vi "Format Errors.vi"(8 "error in (no error)":errorcluster[](array[cluster]), 11 "Channel in":refnum<class "Channel.lvclass">) -> (0 "error out":errorcluster, 3 "Channel out":refnum<class "Channel.lvclass">)   [LabVIEW 2015, in "Channel.lvclass"]
uses:
  Channel.lvclass
  Channel.lvclass/Channel.ctl
  <vilib>/regexp/Match Regular Expression.xnode
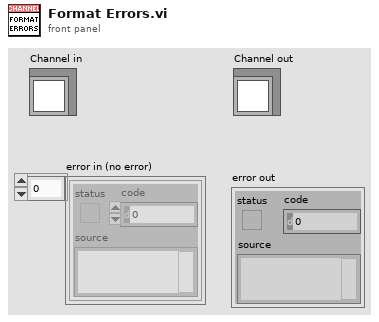
[diagram p1: front panel]
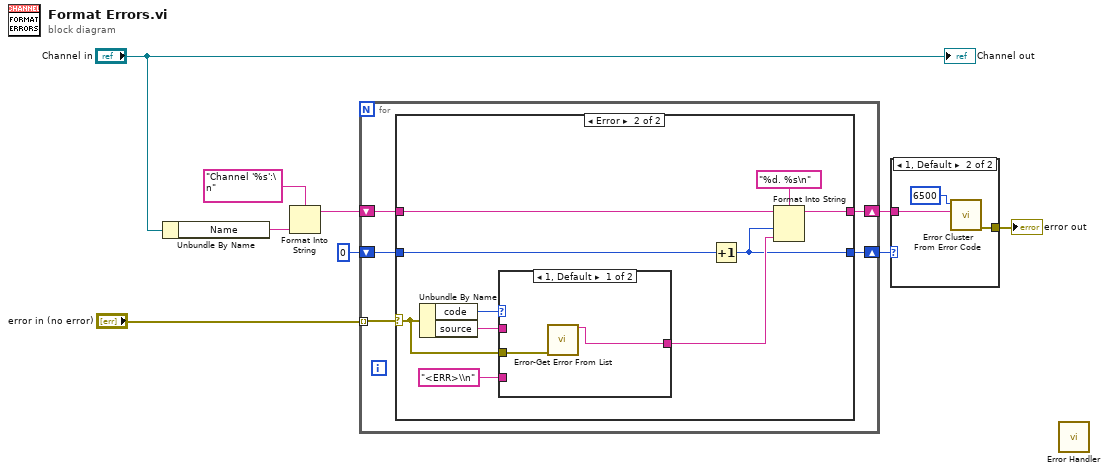
[diagram p0: block diagram]
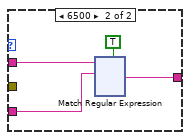
[diagram p4: hidden frame]
diagram:
  n1 = Unbundle By Name("Channel in") -> ("Name"=w6:string)
  n2 = Format Into String(format string="Channel '%s':\n", w6) -> (resulting string=w4:string)  [unwired: 2 in, 1 out]
  n3 = for {
    tunnel: "error in (no error)" -> [w12] mode=indexing
    shift-right: [w13] -> w3
    shift-left: w4 -> [w14]
    shift-right: [w11] -> w1
    shift-left: 0 -> [w10]
    n4 = case shown="Error" w12 {
      selector: w12 -> [_ w17]
      tunnel: w14 -> [w16 w26]
      tunnel: [w16 w25] -> w13
      tunnel: [w15 w19] -> w11
      tunnel: w10 -> [w15 w20]
      frame No Error {
      }
      frame Error {
        n5 = Unbundle By Name(w17) -> ("code"=w18:i32, "source"=w22:string)
        n6 = case shown="1, Default" w18 {
          tunnel: "<ERR>\\n" ("regular expression") -> [_ w31]
          tunnel: w22 -> [_ w30]
          tunnel: [w27 w29] -> w21
          tunnel: w17 -> [w28 _]
          frame 1, Default {
            n7 = call "Error-Get Error From List.vi"("error IO"=w28) -> ("Description"=w27:string)  [unwired: 11 in, 3 out]
          }
          frame 6500 {
            n8 = xnode "Match Regular Expression"("input string"=w30, "regular expression"=w31, "multiline? (F)"=TRUE) -> ("after match"=w29:string)  [unwired: 3 in, 4 out]
          }
        }
        n9 = Increment(x=w20) -> (x+1=w19:i32)
        n10 = Format Into String(format string="%d. %s\n", initial string=w26, w19, w21) -> (resulting string=w25:string)  [unwired: 1 in, 1 out]
      }
    }
  }
  n11 = case shown="1, Default" w1 {
    tunnel: [_ w149] -> w8
    tunnel: w3 -> [_ w148]
    frame 0 {
    }
    frame 1, Default {
      n12 = call <vilib>:"Error Cluster From Error Code.vi"("error message (\"\")"=w148, "error code (0)"=6500) -> ("error out"=w149:errorcluster)  [unwired: 7 in]
    }
  }
  "error out" <- w8
  n13 = call "Error Handler.vi"() -> ()  [unwired: 14 in, 2 out]
  "Channel out" <- "Channel in"
